vi "ControllerIdentification.vi"() -> ()   [LabVIEW 2014]
panel:
  out "Identification":string
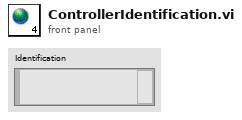
[diagram p1: front panel]
diagram:
